vi "NET_Compressor.vi"(8 "Read(F) Write(T)":bool, 11 "Compressor  In":T1) -> (3 "Compressor Out":T1)   [LabVIEW 2016]
uses:
  TypeDef/Cluster_Compressor.ctl
  <vilib>/Rock Robotics/Network Tables/NT Read Boolean Array.vi
  <vilib>/Rock Robotics/Network Tables/NT Write Boolean Array.vi
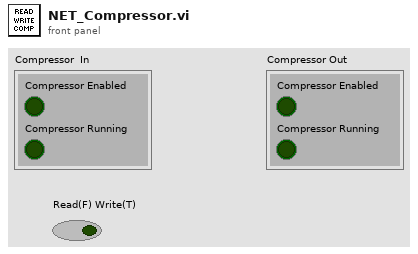
[diagram p1: front panel]
types:
  T1 = typedef "Cluster_Compressor.ctl" = cluster{"Compressor Running":bool, "Compressor Enabled":bool}
  T2 = cluster{"Boolean Array[0]":bool, "Boolean Array[1]":bool}
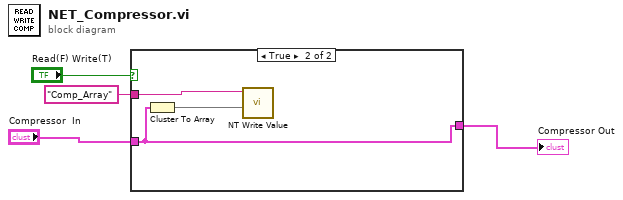
[diagram p0: block diagram]
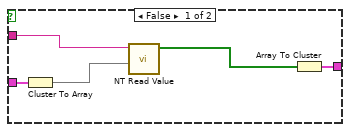
[diagram p2: hidden frame]
diagram:
  n1 = case shown="True" "Read(F) Write(T)" {
    tunnel: "Compressor  In" -> [w8 w10]
    tunnel: "Comp_Array" ("Name") -> [w9 w11]
    tunnel: [w5 w10] -> w1
    frame False {
      n2 = Cluster To Array(cluster=w8) -> (array=w7:bool[])
      n3 = call-poly <vilib>:"NT Read Value.vi"("Default Value"=w7, "Name"=w9) -> ("Boolean Array"=w6:bool[])  [unwired: 8 in, 1 out]
      n4 = Array To Cluster(array=w6) -> (cluster=w5:T2)
    }
    frame True {
      n5 = Cluster To Array(cluster=w10) -> (array=w12:bool[])
      n6 = call-poly <vilib>:"NT Write Value.vi"("Boolean Array"=w12, "Name"=w11) -> ()  [unwired: 9 in, 1 out]
    }
  }
  "Compressor Out" <- w1
